vi "FPS_Counter.vi"(3 "Array in":u32[](array[numeric])) -> (0 "Array out":u32[](array[numeric]), 1 "Numeric":dbl)   [LabVIEW 2016]
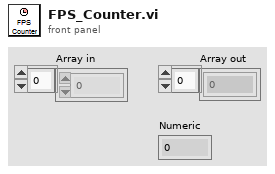
[diagram p1: front panel]
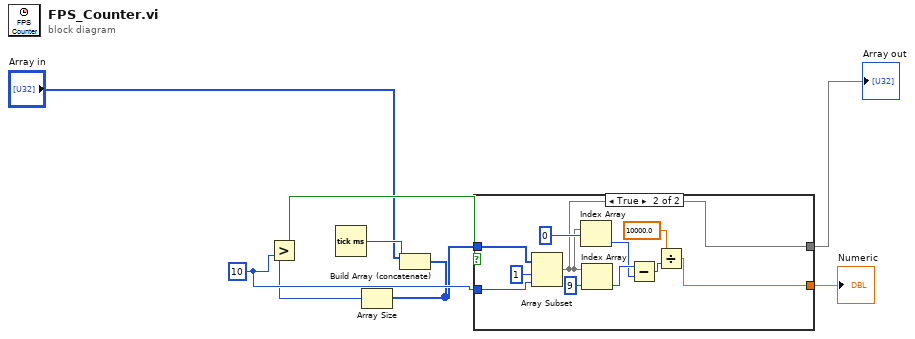
[diagram p0: block diagram]
diagram:
  w5 = 10 ("y")
  n1 = Tick Count (ms)() -> (millisecond timer value=w7:u32)
  n2 = Build Array (concatenate)("Array in", w7) -> (w4:u32[])
  n3 = Array Size(array=w4) -> (size(s)=w2:i32)
  n4 = Greater?(x=w2, y=w5) -> (0:w3:bool)
  n5 = case shown="True" w3 {
    tunnel: w4 -> [w9 w13]
    tunnel: w5 -> [_ w19]
    tunnel: [w9 w11] -> w6
    tunnel: [_ w10] -> w8
    frame False {
    }
    frame True {
      n6 = Array Subset(array=w13, index=1, length=w19) -> (w11:u32[])
      n7 = Index Array(array=w11, index=0) -> (element=w16:u32)
      n8 = Index Array(array=w11, index=9) -> (element=w17:u32)
      n9 = Subtract(x=w17, y=w16) -> (x-y=w15:u32)
      n10 = Divide(x=10000.0, y=w15) -> (x/y=w10:dbl)
    }
  }
  "Numeric" <- w8
  "Array out" <- w6
